vi "SetupFile_GetElapsedDuration.vi"(11 "Path":path) -> (3 "date/time string":string)   [LabVIEW 2020]
uses:
  <vilib>/Utility/file.llb/Read Delimited Spreadsheet (string).vi
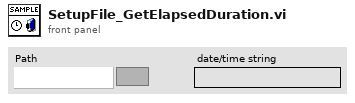
[diagram p1: front panel]
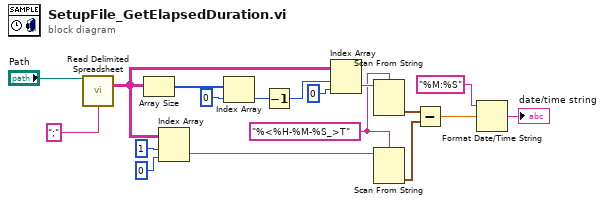
[diagram p0: block diagram]
diagram:
  w12 = "%<%H-%M-%S_>T" ("time format string (%c)")
  n1 = call-poly <vilib>:"Read Delimited Spreadsheet.vi"("file path (dialog if empty)"="Path", "delimiter (\\t)"=";" ("delimiter (\\t)")) -> ("all rows"=w7:string[][])  [unwired: 8 in, 5 out]
  n2 = Array Size(array=w7) -> (size(s)=w8:i32[])
  n3 = Index Array(array=w7, index (row)=1, index (col)=0 ("disabled index (col)")) -> (element=w11:string)
  n4 = Index Array(array=w8, index=0) -> (element=w10:i32)
  n5 = Decrement(x=w10) -> (x-1=w1:i32)
  n6 = Index Array(array=w7, index (row)=w1, index (col)=0 ("disabled index (col)")) -> (element=w13:string)
  n7 = Scan From String(format string=w12, input string=w13) -> (output 1=w14:timestamp)  [unwired: 3 in, 3 out]
  n8 = Scan From String(format string=w12, input string=w11) -> (output 1=w15:timestamp)  [unwired: 3 in, 3 out]
  n9 = Subtract(x=w14, y=w15) -> (x-y=w17:dbl)
  n10 = Format Date/Time String(time format string (%c)="%M:%S", seconds (now)=w17) -> (date/time string=→"date/time string":string)  [unwired: 1 in]
